vi "Day07-01.vi"() -> ()   [LabVIEW 2021]
uses:
  <vilib>/DAQmx/write.llb/DAQmx Write (Analog Wfm 1Chan NSamp).vi
  <vilib>/DAQmx/create/channels.llb/DAQmx Create Channel (AO-Voltage-Basic).vi
  <vilib>/DAQmx/configure/timing.llb/DAQmx Timing (Use Waveform).vi
  <vilib>/DAQmx/miscellaneous.llb/DAQmx Fill In Error Info.vi
  <vilib>/DAQmx/configure/trigger.llb/DAQmx Start Trigger (Analog Edge).vi
  <vilib>/DAQmx/write.llb/DAQmx Write (Analog DBL 1Chan 1Samp).vi
  <vilib>/DAQmx/read.llb/DAQmx Read (Analog Wfm 1Chan NSamp).vi
  <vilib>/DAQmx/create/channels.llb/DAQmx Create Channel (AI-Voltage-Basic).vi
  <vilib>/DAQmx/configure/timing.llb/DAQmx Timing (Sample Clock).vi
  <vilib>/DAQmx/configure/trigger.llb/DAQmx Start Trigger (Digital Edge).vi
  <vilib>/measure/NI_MABase.lvlib
panel:
  in  "정지 3":bool
  out "웨이브폼 그래프 2":waveform(dbl)(graph)
  out "웨이브폼 그래프":waveform(dbl)(graph)
  in  "정지 2":bool
  in  "data 2":dbl caption="데이터" format="%0.2f"
  in  "정지":bool
  out "data":waveform(dbl)(graph) caption="데이터"
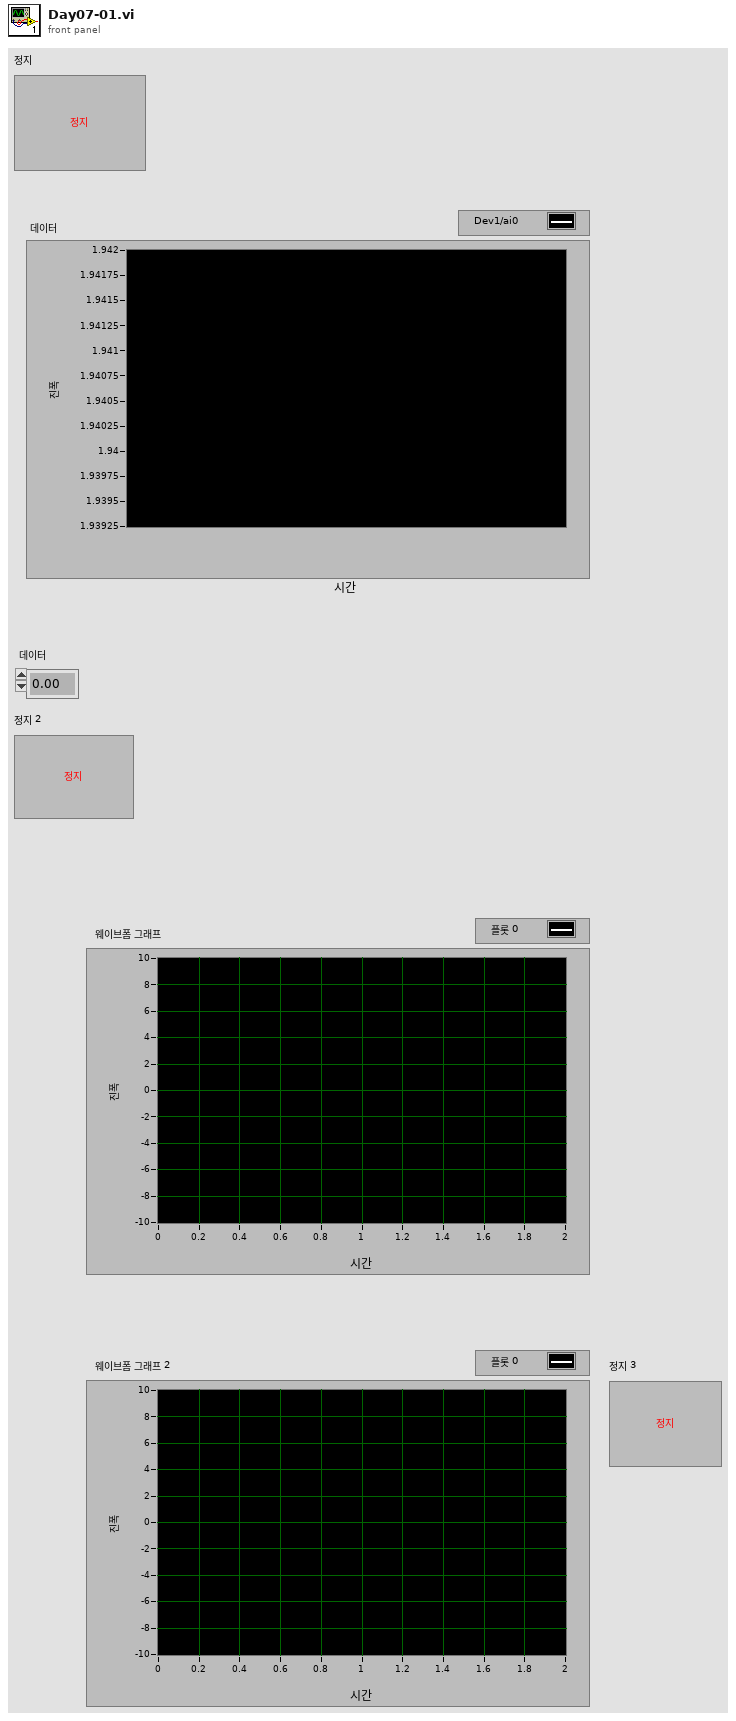
[diagram p1: front panel]
types:
  T1 = enum16{"Sine Wave", "Triangle Wave", "Square Wave", "Sawtooth Wave"}
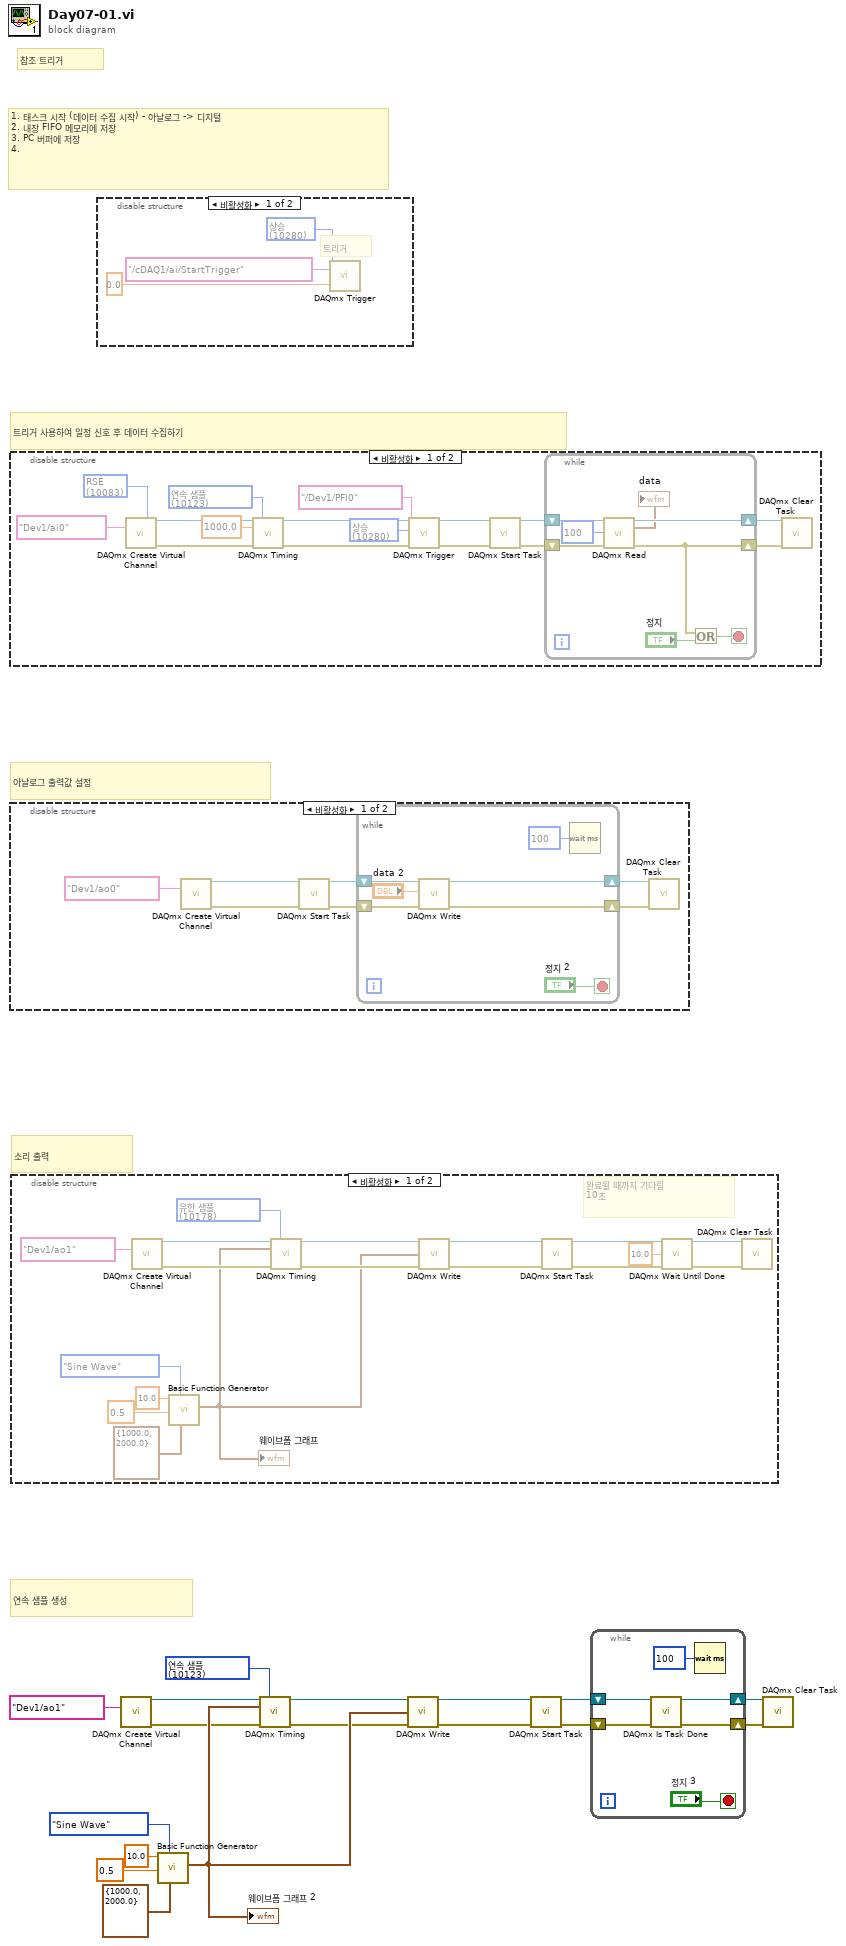
[diagram p0: block diagram]
diagram:
  w12 = 10123 items=["유한 샘플"=10178, "연속 샘플"=10123, "하드웨어 타이밍에 의한 단일 포인트"=12522] ("sample mode")
  # "연속 샘플 생성"
  # "소리 출력"
  # "아날로그 출력값 설정"
  # "트리거 사용하여 일정 신호 후 데이터 수집하기"
  # "참조 트리거"
  # "1. 태스크 시작 (데이터 수집 시작) - 아날로그 -> 디지털\n2. 내장 FIFO 메모리에 저장\n3. PC 버퍼에 저장\n4."
  n1 = disable-structure shown="비활성화" {
    frame Disabled {
      w19 = 10083 items=["기본"=-1, "RSE"=10083, "NRSE"=10078, "차동"=10106, "유사 차동"=12529] ("input terminal configuration")
      w20 = 10280 items=["상승"=10280, "하강"=10171] ("edge")
      w22 = 10123 items=["유한 샘플"=10178, "연속 샘플"=10123, "하드웨어 타이밍에 의한 단일 포인트"=12522] ("sample mode")
      n2 = call-poly <vilib>:"DAQmx Create Virtual Channel.vi"("input terminal configuration"=w19, "physical channels"=tag "Dev1/ai0") -> ("task out"=w33:refnum<k21>, "error out"=w32:errorcluster)  [unwired: 12 in]
      n3 = call-poly <vilib>:"DAQmx Timing.vi"("task/channels in"=w33, "sample mode"=w22, "rate"=1000.0, "error in"=w32) -> ("task out"=w31:refnum<k21>, "error out"=w30:errorcluster)  [unwired: 10 in]
      n4 = call-poly <vilib>:"DAQmx Trigger.vi"("task/channels in"=w31, "source"=tag "/Dev1/PFI0", "edge"=w20, "error in"=w30) -> ("task out"=w29:refnum<k21>, "error out"=w28:errorcluster)  [unwired: 10 in]
      n5 = call <vilib>:"DAQmx Start Task.vi"("task/channels in"=w29, "error in"=w28) -> ("task out"=w27:refnum<k21>, "error out"=w26:errorcluster)  [unwired: 12 in]
      n6 = while {
        shift-right: [w39] -> w25
        shift-left: w27 -> [w41]
        shift-right: [w36] -> w24
        shift-left: w26 -> [w40]
        stop <- w34 stop-if-true
        n7 = call-poly <vilib>:"DAQmx Read.vi"("task/channels in"=w41, "number of samples per channel"=100, "error in"=w40) -> ("task out"=w39:refnum<k21>, "data"=→"data":waveform(dbl), "error out"=w36:errorcluster)  [unwired: 10 in]
        n8 = Or(x=w36, y="정지") -> (x .or. y?=w34:bool)
      }
      n9 = call <vilib>:"DAQmx Clear Task.vi"("task in"=w25, "error in"=w24) -> ()  [unwired: 13 in, 1 out]
    }
    frame Enabled {
    }
  }
  n10 = disable-structure shown="비활성화" {
    frame Disabled {
      n11 = call-poly <vilib>:"DAQmx Create Virtual Channel.vi"("physical channels"=tag "Dev1/ao0") -> ("task out"=w48:refnum<k21>, "error out"=w47:errorcluster)  [unwired: 13 in]
      n12 = call <vilib>:"DAQmx Start Task.vi"("task/channels in"=w48, "error in"=w47) -> ("task out"=w46:refnum<k21>, "error out"=w45:errorcluster)  [unwired: 12 in]
      n13 = while {
        shift-right: [w53] -> w44
        shift-left: w46 -> [w55]
        shift-right: [w52] -> w43
        shift-left: w45 -> [w54]
        stop <- "정지 2" stop-if-true
        n14 = call-poly <vilib>:"DAQmx Write.vi"("task/channels in"=w55, "data"="data 2", "error in"=w54) -> ("task out"=w53:refnum<k21>, "error out"=w52:errorcluster)  [unwired: 10 in, 1 out]
        n15 = Wait (ms)(milliseconds to wait=u32 100 ("대기 시간 (ms)")) -> ()  [unwired: 1 out]
      }
      n16 = call <vilib>:"DAQmx Clear Task.vi"("task in"=w44, "error in"=w43) -> ()  [unwired: 13 in, 1 out]
    }
    frame Enabled {
    }
  }
  n17 = disable-structure shown="비활성화" {
    frame Disabled {
      w62 = 10178 items=["유한 샘플"=10178, "연속 샘플"=10123, "하드웨어 타이밍에 의한 단일 포인트"=12522] ("sample mode")
      # "완료될 때까지 기다림\n10초"
      n18 = call-poly <vilib>:"DAQmx Create Virtual Channel.vi"("physical channels"=tag "Dev1/ao1") -> ("task out"=w73:refnum<k21>, "error out"=w72:errorcluster)  [unwired: 13 in]
      n19 = call <vilib>:"Basic Function Generator.vi"("sampling info"=cluster{"Fs":dbl, "#s":dbl} {"Fs"=1000.0, "#s"=2000.0}, "signal type"=T1."Sine Wave", "amplitude"=0.5, "frequency"=10.0) -> ("signal out"=w57:waveform(dbl))  [unwired: 5 in, 2 out]
      "웨이브폼 그래프" <- w57
      n20 = call-poly <vilib>:"DAQmx Timing.vi"("task/channels in"=w73, "sample mode"=w62, "waveform"=w57, "error in"=w72) -> ("task out"=w71:refnum<k21>, "error out"=w70:errorcluster)  [unwired: 10 in]
      n21 = call-poly <vilib>:"DAQmx Write.vi"("task/channels in"=w71, "data"=w57, "error in"=w70) -> ("task out"=w69:refnum<k21>, "error out"=w68:errorcluster)  [unwired: 10 in, 1 out]
      n22 = call <vilib>:"DAQmx Start Task.vi"("task/channels in"=w69, "error in"=w68) -> ("task out"=w67:refnum<k21>, "error out"=w66:errorcluster)  [unwired: 12 in]
      n23 = call <vilib>:"DAQmx Wait Until Done.vi"("task/channels in"=w67, "timeout (sec)"=10.0, "error in"=w66) -> ("task out"=w65:refnum<k21>, "error out"=w64:errorcluster)  [unwired: 11 in]
      n24 = call <vilib>:"DAQmx Clear Task.vi"("task in"=w65, "error in"=w64) -> ()  [unwired: 13 in, 1 out]
    }
    frame Enabled {
    }
  }
  n25 = disable-structure shown="비활성화" {
    frame Disabled {
      w75 = 10280 items=["상승"=10280, "하강"=10171] ("edge")
      # "트리거"
      n26 = call-poly <vilib>:"DAQmx Trigger.vi"("source"=tag "/cDAQ1/ai/StartTrigger", "slope"=w75, "level"=0.0) -> ()  [unwired: 11 in, 2 out]
    }
    frame Enabled {
    }
  }
  n27 = call-poly <vilib>:"DAQmx Create Virtual Channel.vi"("physical channels"=tag "Dev1/ao1") -> ("task out"=w1:refnum<k21>, "error out"=w2:errorcluster)  [unwired: 13 in]
  n28 = call <vilib>:"Basic Function Generator.vi"("sampling info"=cluster{"Fs":dbl, "#s":dbl} {"Fs"=1000.0, "#s"=2000.0}, "signal type"=T1."Sine Wave", "amplitude"=0.5, "frequency"=10.0) -> ("signal out"=w17:waveform(dbl))  [unwired: 5 in, 2 out]
  "웨이브폼 그래프 2" <- w17
  n29 = call-poly <vilib>:"DAQmx Timing.vi"("task/channels in"=w1, "sample mode"=w12, "waveform"=w17, "error in"=w2) -> ("task out"=w3:refnum<k21>, "error out"=w4:errorcluster)  [unwired: 10 in]
  n30 = call-poly <vilib>:"DAQmx Write.vi"("task/channels in"=w3, "data"=w17, "error in"=w4) -> ("task out"=w5:refnum<k21>, "error out"=w6:errorcluster)  [unwired: 10 in, 1 out]
  n31 = call <vilib>:"DAQmx Start Task.vi"("task/channels in"=w5, "error in"=w6) -> ("task out"=w7:refnum<k21>, "error out"=w8:errorcluster)  [unwired: 12 in]
  n32 = while {
    shift-right: [w82] -> w10
    shift-left: w8 -> [w80]
    shift-right: [w81] -> w9
    shift-left: w7 -> [w79]
    stop <- "정지 3" stop-if-true
    n33 = call <vilib>:"DAQmx Is Task Done.vi"("task/channels in"=w79, "error in"=w80) -> ("task out"=w81:refnum<k21>, "error out"=w82:errorcluster)  [unwired: 11 in, 1 out]
    n34 = Wait (ms)(milliseconds to wait=u32 100 ("대기 시간 (ms)")) -> ()  [unwired: 1 out]
  }
  n35 = call <vilib>:"DAQmx Clear Task.vi"("task in"=w9, "error in"=w10) -> ()  [unwired: 13 in, 1 out]
